vi "setFPGAReference.vi"(10 "FPGAReference":refnum<k20>, 11 "ModbusIRQs in":refnum<class "ModbusIRQs.lvclass">) -> (3 "ModbusIRQs out":refnum<class "ModbusIRQs.lvclass">)   [LabVIEW 2016, in "ModbusIRQs.lvclass"]
uses:
  ModbusIRQs.lvclass
  ModbusIRQs.lvclass/ModbusIRQs.ctl
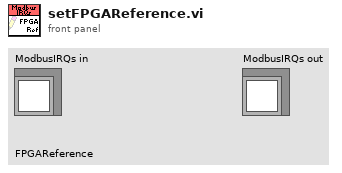
[diagram p1: front panel]
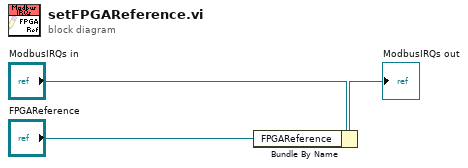
[diagram p0: block diagram]
diagram:
  n1 = Bundle By Name(cluster="ModbusIRQs in", "FPGAReference"="FPGAReference") -> (→"ModbusIRQs out":refnum<class "ModbusIRQs.lvclass">)
